vi "F11xx_FileMerger_V1.vi"() -> ()   [LabVIEW 2018]
uses:
  <vilib>/Utility/file.llb/Read From Spreadsheet File (string).vi
  <vilib>/Utility/file.llb/Write To Spreadsheet File (string).vi
panel:
  out "Array 4":i32[](array[numeric])=[37, 36, 36, 36, 36, 36, 36, 36, 36, 36, 36, 36, 36, 36, 36, 36, 36, 36, 36, 36, 36, 36]
  out "Array 3":bool[](array[boolean])
  out "Array 2":string[](array[string])=["10", "11", "12", "13", "14", "15", "16", "17", "18", "19", "1", "20", "21", "22", "2", "3", "4", "5", "6", "7", "8", "9"]
  out "Boolean":bool
  in  "Write to File":bool
  in  "Folder":path=path "\\\\Corpmxl0251xct\\c/IdtATE/Results/Loadbrd _r2_firstlook_F1150_080811/EvKit Plunge"
  in  "Target File":path=path "\\\\Corpmxl0251xct\\c/IdtATE/Results/Loadbrd _r2_firstlook_F1150_080811/EvKit Plunge/Loadbrd _r2_firstlook_F1150_080811_SN_1Thru22.csv"
  in  "offset (0) 2":i32=40
  in  "offset (0)":i32=11
  out "Array":string[](array[string])=["9", "9", "9", "9", "9", "9", "9", "9", "9", "9", "9", "9", "9", "9", "9", "9", "9", "9", "9", "9", "9", "9", "9", "9", "9", "9", "9", "9", "9", "9", "9", "9", "9", "9", "9", "9"]
  out "element":i32=36
  out "filenames":string[](array[string])=["Loadbrd _r2_firstlook_F1150_080811_SN_1-10_151403.csv", "Loadbrd _r2_firstlook_F1150_080811_SN_1-11_152349.csv", "Loadbrd _r2_firstlook_F1150_080811_SN_1-12_153322.csv", "Loadbrd _r2_firstlook_F1150_080811_SN_1-13_154231.csv", "Loadbrd _r2_firstlook_F1150_080811_SN_1-14_155132.csv", "Loadbrd _r2_firstlook_F1150_080811_SN_1-15_160102.csv", "Loadbrd _r2_firstlook_F1150_080811_SN_1-16_161750.csv", "Loadbrd _r2_firstlook_F1150_080811_SN_1-17_162638.csv", "Loadbrd _r2_firstlook_F1150_080811_SN_1-18_163501.csv", "Loadbrd _r2_firstlook_F1150_080811_SN_1-19_164508.csv", "Loadbrd _r2_firstlook_F1150_080811_SN_1-1_134125.csv", "Loadbrd _r2_firstlook_F1150_080811_SN_1-20_165401.csv", "Loadbrd _r2_firstlook_F1150_080811_SN_1-21_170335.csv", "Loadbrd _r2_firstlook_F1150_080811_SN_1-22_171202.csv", "Loadbrd _r2_firstlook_F1150_080811_SN_1-2_135257.csv", "Loadbrd _r2_firstlook_F1150_080811_SN_1-3_140438.csv", "Loadbrd _r2_firstlook_F1150_080811_SN_1-4_141457.csv", "Loadbrd _r2_firstlook_F1150_080811_SN_1-5_142448.csv", "Loadbrd _r2_firstlook_F1150_080811_SN_1-6_143320.csv", "Loadbrd _r2_firstlook_F1150_080811_SN_1-7_144223.csv", "Loadbrd _r2_firstlook_F1150_080811_SN_1-8_145159.csv", "Loadbrd _r2_firstlook_F1150_080811_SN_1-9_150415.csv"]
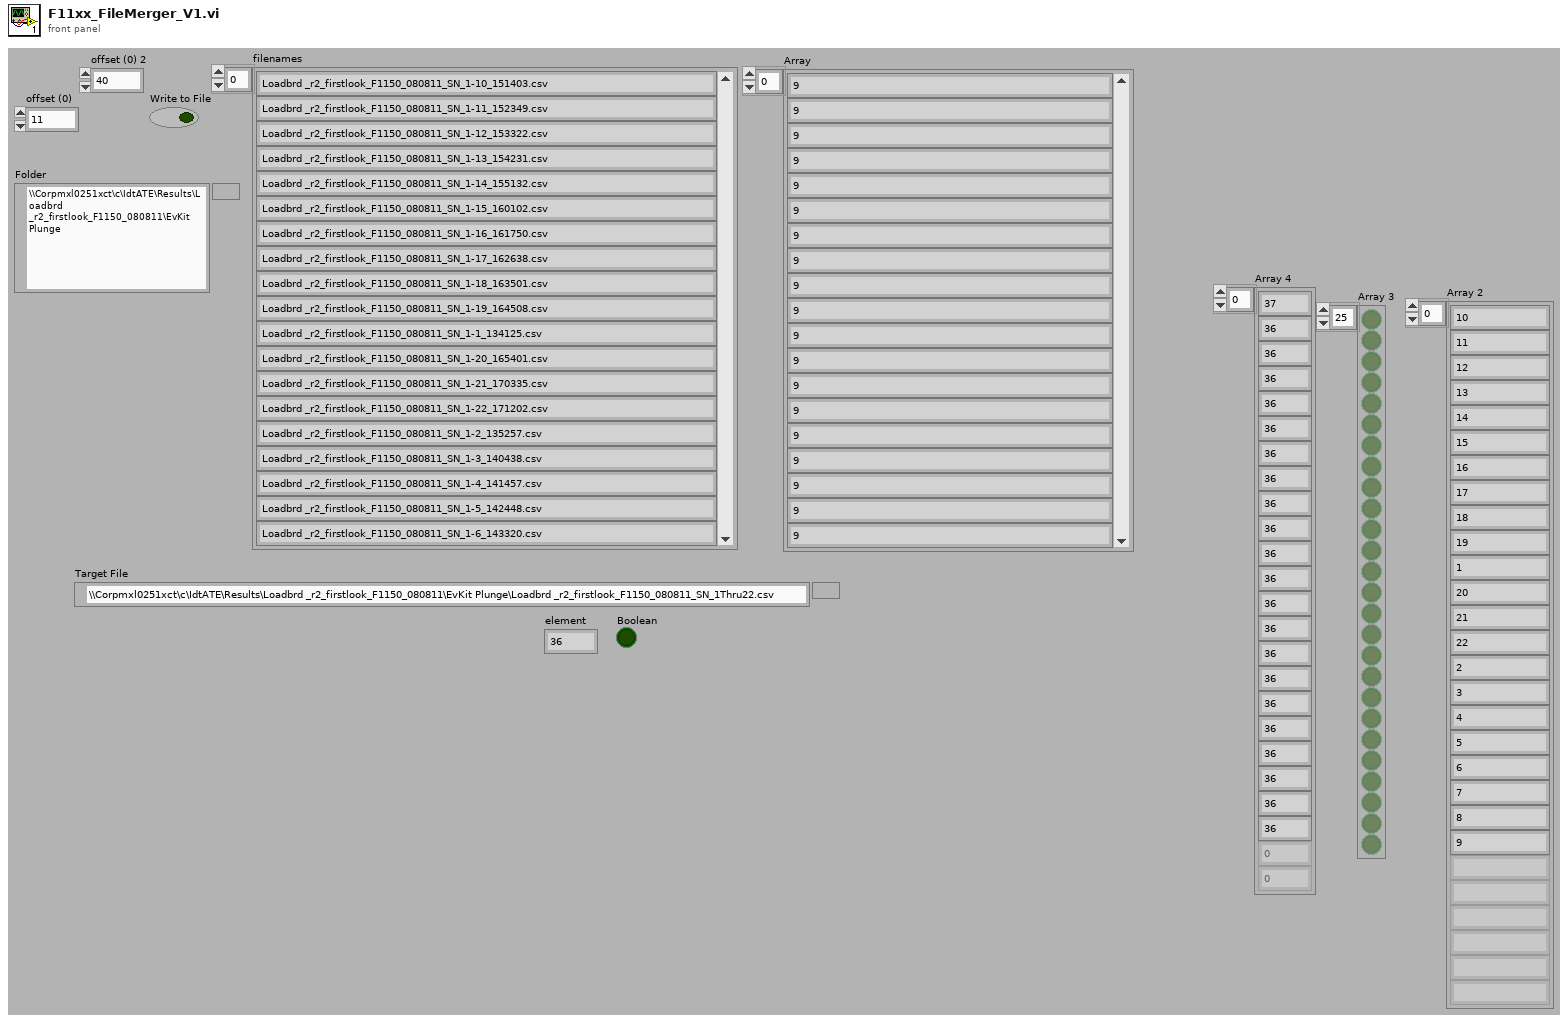
[diagram p1: front panel]
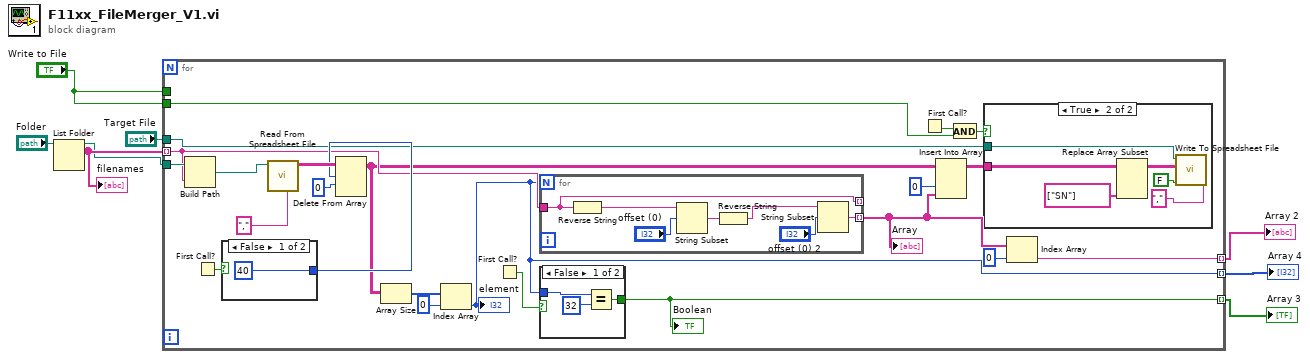
[diagram p0: block diagram]
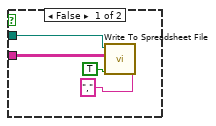
[diagram p3: hidden frame]
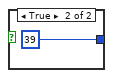
[diagram p4: hidden frame]
diagram:
  n1 = List Folder(path="Folder") -> (path out=w6:path, filenames=w7:string[])  [unwired: 3 in, 2 out]
  "filenames" <- w7
  n2 = for {
    tunnel: w7 -> [w24] mode=indexing
    tunnel: w6 -> [w28]
    tunnel: "Target File" -> [w21]
    tunnel: "Write to File" -> [_]
    tunnel: "Write to File" -> [w9]
    tunnel: [w13] -> w3 mode=indexing
    tunnel: [w12] -> w2 mode=indexing
    tunnel: [w11] -> w1 mode=indexing
    n3 = Build Path(base path=w28, name or relative path=w24) -> (appended path=w27:path)
    n4 = First Call?() -> (First Call?: T/F=w22:bool)
    n5 = case shown="False" w22 {
      tunnel: [40 ("length") 39 ("length")] -> w30
      frame False {
      }
      frame True {
      }
    }
    n6 = call-poly <vilib>:"Read From Spreadsheet File.vi"("delimiter (\\t)"="," ("delimiter (\\t)"), "file path (dialog if empty)"=w27) -> ("all rows"=w31:string[][])  [unwired: 5 in, 4 out]
    n7 = Delete From Array(array=w31, length=w30, index (row)=0) -> (array with subset deleted=w23:string[][])  [unwired: 1 in, 1 out]
    n8 = Array Size(array=w23) -> (size(s)=w26:i32[])
    n9 = Index Array(array=w26, index=0) -> (element=w11:i32)
    "element" <- w11
    n10 = First Call?() -> (First Call?: T/F=w16:bool)
    n11 = for {
      N: w11 -> [_]
      tunnel: [w52] -> _ mode=indexing
      tunnel: w24 -> [w52]
      tunnel: [w48] -> w15 mode=indexing
      n12 = Reverse String(1:w52) -> (0:w51:string)
      n13 = String Subset(string=w51, offset (0)="offset (0)") -> (substring=w53:string)  [unwired: 1 in]
      n14 = Reverse String(1:w53) -> (0:w49:string)
      n15 = String Subset(string=w49, offset (0)="offset (0) 2") -> (substring=w48:string)  [unwired: 1 in]
    }
    "Array" <- w15
    n16 = case shown="False" w16 {
      tunnel: w11 -> [w34 _]
      tunnel: [w32 _] -> w12
      frame False {
        n17 = Equal?(x=w34, y=32) -> (x = y?=w32:bool)
      }
      frame True {
      }
    }
    "Boolean" <- w12
    n18 = First Call?() -> (First Call?: T/F=w18:bool)
    n19 = Insert Into Array(array=w23, index (col)=0 ("disabled index (col)"), new element=w15) -> (w19:string[][])  [unwired: 1 in]
    n20 = And(x=w18, y=w9) -> (x .and. y?=w10:bool)
    n21 = case shown="True" w10 {
      tunnel: w19 -> [w38 w41]
      tunnel: w21 -> [w35 w42]
      frame False {
        n22 = call-poly <vilib>:"Write To Spreadsheet File.vi"("delimiter (\\t)"="," ("delimiter (\\t)"), "append to file? (new file:F)"=TRUE, "2D data"=w38, "file path (dialog if empty)"=w35) -> ()  [unwired: 4 in, 1 out]
      }
      frame True {
        n23 = Replace Array Subset(array=w41, new element=string[] ["SN"] ("new element/subarray")) -> (w39:string[][])  [unwired: 2 in]
        n24 = call-poly <vilib>:"Write To Spreadsheet File.vi"("delimiter (\\t)"="," ("delimiter (\\t)"), "append to file? (new file:F)"=FALSE, "2D data"=w39, "file path (dialog if empty)"=w42) -> ()  [unwired: 4 in, 1 out]
      }
    }
    n25 = Index Array(array=w15, index=0) -> (element=w13:string)
  }
  "Array 2" <- w3
  "Array 3" <- w2
  "Array 4" <- w1
